vi "Copilot Speech.vi"(8 "error in (no error)":errorcluster, 11 "TEXT TO BE SPOKEN":string="LabVIEW is the greatest software ever to be created. Next to the spork, there is no better invention!!") -> (0 "error out":errorcluster)   [LabVIEW 2014]
doc: "This VI speaks in the default windows voice."
panel:
  in  "SpeechLib.ISpeechVoice":refnum<k7>
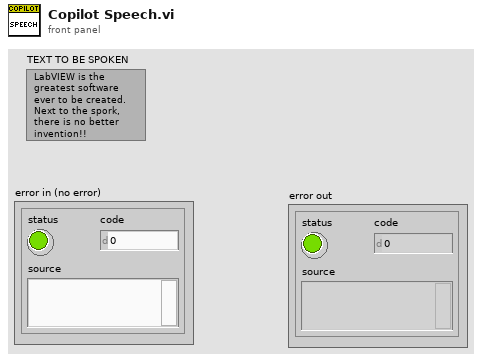
[diagram p1: front panel]
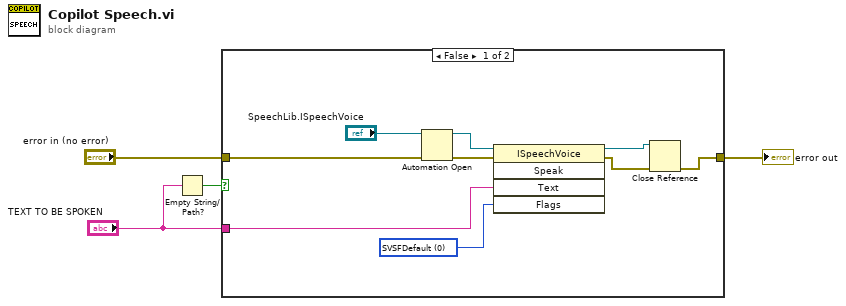
[diagram p0: block diagram]
diagram:
  n1 = Empty String/Path?(string/path="TEXT TO BE SPOKEN") -> (empty?=w1:bool)
  n2 = case shown="False" w1 {
    tunnel: [w7 w14] -> w4
    tunnel: "error in (no error)" -> [w6 w14]
    tunnel: "TEXT TO BE SPOKEN" -> [w5 _]
    frame False {
      w12 = 0 items=["SVSFDefault"=0, "SVSFlagsAsync"=1, "SVSFPurgeBeforeSpeak"=2, "SVSFIsFilename"=4, "SVSFIsXML"=8, "SVSFIsNotXML"=16, "SVSFPersistXML"=32, "SVSFNLPSpeakPunc, SVSFNLPMask"=64, "SVSFVoiceMask"=127, "SVSFUnusedFlags"=-128] ("Flags")
      n3 = Automation Open(error in (no error)=w6, Automation Refnum="SpeechLib.ISpeechVoice") -> (Automation Refnum=w10:refnum<k7>, error out=w11:errorcluster)  [unwired: 2 out]
      n4 = invoke class="ISpeechVoice" method="Speak"(reference=w10, error in=w11, "Text"=w5, "Flags"=w12) -> (reference out=w8:refnum<k7>, error out=w9:errorcluster)  [unwired: 1 in, 3 out]
      n5 = Close Reference(reference=w8, error in (no error)=w9) -> (error out=w7:errorcluster)
    }
    frame True {
      # "Empty string. do nothing"
    }
  }
  "error out" <- w4
